vi "Cache Master Danielsson.vi"(8 "error in (no error)":errorcluster, 11 "Image In":T1) -> (0 "error out":errorcluster, 3 "Image out":T1)   [LabVIEW 2013]
doc: "This vi uses a Daniellson tranfomation of the drop binary image followed by a threshold to shrink the diameter of the drop mask. Any point originally part of the mask that is within \"pixels to shrink\" of the boarder is removed from the drop mask out."
uses:
  <vilib>/vision/NI_Vision_Development_Module.lvlib
  Project Vis/Image Processing/Image processing type defs/Image spaces (processing) names enum.ctl
  <vilib>/vision/Image Controls.llb/IMAQ Image.ctl
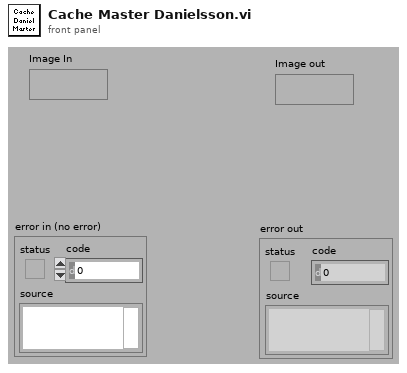
[diagram p1: front panel]
types:
  T1 = typedef "IMAQ Image.ctl" = refnum<image>
  T2 = typedef "Image spaces (processing) names enum.ctl" = enum16{"Master - HSL", "UUT - HSL", "Master binary 0 - U8", "Master binary 1 - U8", "Master binary 2 - U8", "Master binary 3 - U8", "Master binary 4 - U8", "Score 0 - U8", "Score 1 - U8", "Score 2 - U8", "Score 3 - U8", "Score 4 - U8", "UUT binary 0 - U8", "UUT binary 1 - U8", "UUT binary 2 - U8", "UUT binary 3 - U8", "UUT binary 4 - U8", "UUT All Colors Mask - U8", "Process 1 - U8", "Process 2 - U8", "Process 1 - SGL", "Mask - U8", "Plate mask - U8", "Master rotation unwrap - U8", "UUT rotation unwrap - U8", "UUT blob 0 - U8", "UUT blob 1 - U8", "UUT blob 2 - U8", "UUT blob 3 - U8", "UUT blob 4 - U8", "Missing color 0 - U8", "Missing color 1 - U8", "Missing color 2 - U8", "Missing color 3 - U8", "Missing color 4 - U8", "Save - RGB", "Master binary 0 D - U8", "Master binary 0 DRaw - U8"}
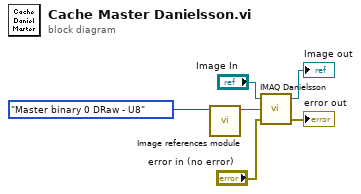
[diagram p0: block diagram]
diagram:
  n1 = call "Image references module.vi"("Image space 1"=Image_spaces_(processing)_names_enum."Master binary 0 DRaw - U8") -> ("Image 1"=w2:T1)  [unwired: 6 in, 4 out]
  n2 = call "IMAQ Danielsson"("error in (no error)"="error in (no error)", "Image Dst"=w2, "Image Src"="Image In") -> ("error out"=→"error out":errorcluster, "Image Dst Out"=→"Image out":T1)  [unwired: 1 in]
